vi "SDCP SMF Receiver and Transmitter - SMF Rx Table.vi"(2 "error in (no error)":errorcluster, 3 "Table reference":refnum<vi>) -> (0 "error out":errorcluster)   [LabVIEW 2020]
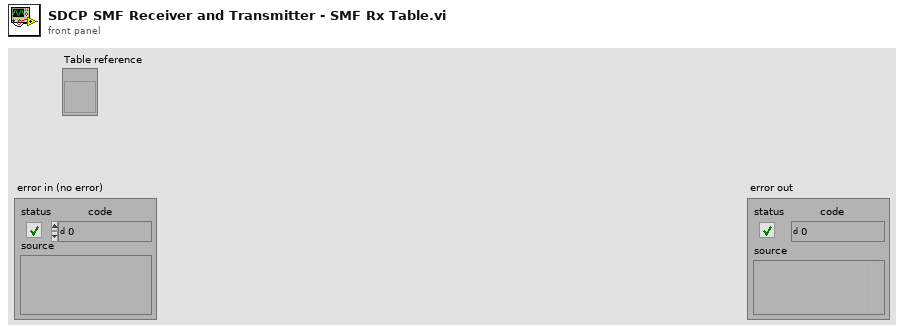
[diagram p1: front panel]
types:
  T1 = typedef "SDCP SMF Receiver and Transmitter - Notifier and Queues.ctl" = cluster{"Trace Queue":refnum<queue>, "Tx - Log Table Queue":refnum<queue>, "Tx - User Queue":refnum<queue>, "Rx - Log Table Queue":refnum<queue>, "Rx - User Queue":refnum<queue>, "Log status Notifier":refnum<notifier>, "Plot Queue":refnum<queue>}
  T2 = typedef "SDCP SMF logger - SMF with timestamp.ctl" = cluster{"Bytes":u8[], "Checksum":bool, "Time (ms)":u32, "Tx/Rx":string}
  T3 = typedef "SDCP - SMF parameter descriptors.ctl" = cluster{"Frame name":string, "Frame ID":i32, "Data type":string, "Start Position":i32, "Length":i32, "Factor":dbl, "Offset":dbl, "Parameter name":string, "Value":string}
  T4 = typedef "SDCP - Log Table - Element.ctl" = cluster{"Data frame":u8[], "Cycle time (ms)":i32, "Count":i32, "Frame ID":i32, "Frame name":string, "Parameter names":string[], "Parameter values":string[]}
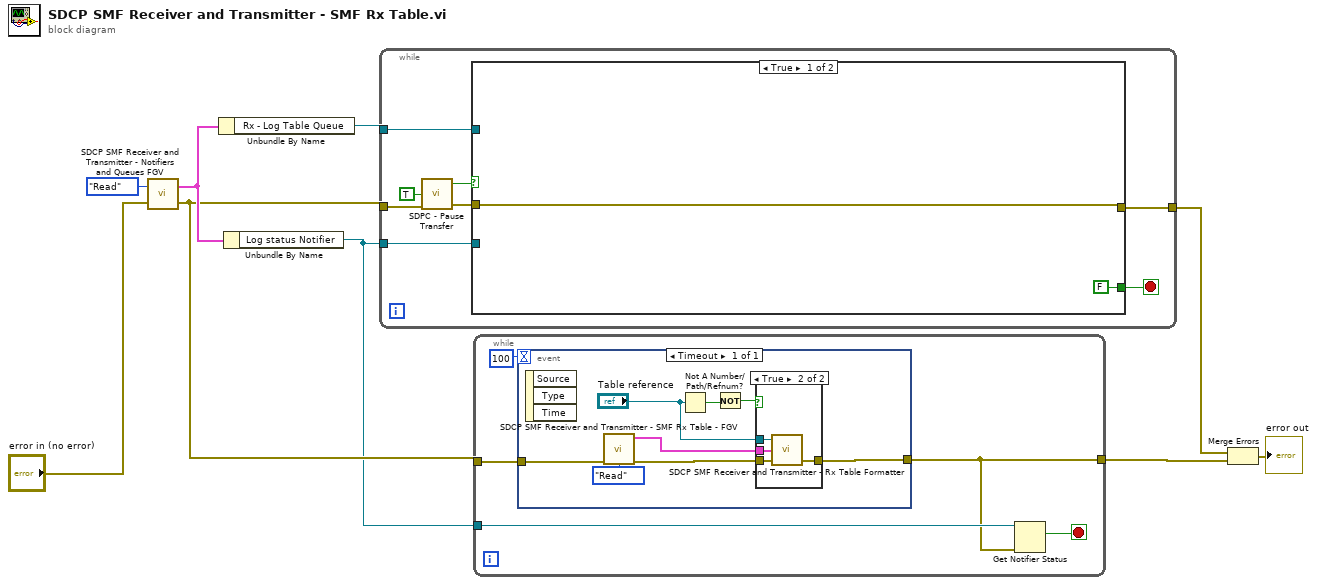
[diagram p0: block diagram]
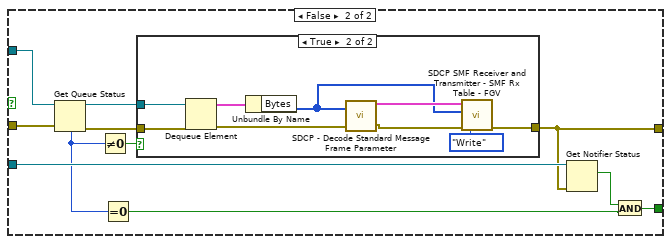
[diagram p3: hidden frame]
diagram:
  n1 = call "SDCP SMF Receiver and Transmitter - Notifiers and Queues FGV.vi"("error in (no error)"="error in (no error)", "Command"=enum16{"Initialize", "Read", "Deinitialize"}."Read") -> ("error out"=w3:errorcluster, "Output"=w6:T1)
  n2 = Unbundle By Name(w6) -> ("Rx - Log Table Queue"=w7:refnum<queue>)
  n3 = Unbundle By Name(w6) -> ("Log status Notifier"=w1:refnum<notifier>)
  n4 = while {
    tunnel: w3 -> [w13]
    tunnel: w7 -> [w15]
    tunnel: w1 -> [w17]
    tunnel: [w16] -> w5
    stop <- w14 stop-if-true
    n5 = call "SDPC - Pause Transfer.vi"("error in (no error)"=w13, "RD/nWR"=TRUE) -> ("error out"=w11:errorcluster, "Transfer paused"=w10:bool)  [unwired: 2 in]
    n6 = case shown="True" w10 {
      tunnel: w17 -> [_ w30]
      tunnel: [w19 w29] -> w16
      tunnel: w15 -> [_ w26]
      tunnel: [FALSE w23] -> w14
      tunnel: w11 -> [w19 w20]
      frame True {
      }
      frame False {
        n7 = Get Queue Status(queue=w26, error in (no error)=w20) -> (queue out=w25:refnum<queue>, error out=w28:errorcluster, # elements in queue=w22:i32)  [unwired: 1 in, 5 out]
        n8 = Not Equal To 0?(x=w22) -> (x != 0?=w27:bool)
        n9 = Equal To 0?(x=w22) -> (x = 0?=w21:bool)
        n10 = case shown="True" w27 {
          tunnel: [w31 w34] -> w29
          tunnel: w28 -> [w31 w33]
          tunnel: w25 -> [_ w32]
          frame False {
          }
          frame True {
            n11 = Dequeue Element(queue=w32, error in (no error)=w33) -> (element=w39:T2, error out=w40:errorcluster)  [unwired: 1 in, 2 out]
            n12 = Unbundle By Name(w39) -> ("Bytes"=w36:u8[])
            n13 = call "SDCP - Decode Standard Message Frame Parameter.vi"("error in (no error)"=w40, "Bytes in"=w36) -> ("error out"=w38:errorcluster, "SMF Parameters out"=w37:T3[])
            n14 = call "SDCP SMF Receiver and Transmitter - SMF Rx Table - FGV.vi"("error in (no error)"=w38, "Command"=enum16{"Reset", "Write", "Read"}."Write", "Bytes in"=w36, "Parameter descriptors"=w37) -> ("error out"=w34:errorcluster)  [unwired: 6 in, 1 out]
          }
        }
        n15 = Get Notifier Status(notifier=w30, error in (no error)=w29) -> (current notification=w24:bool)  [unwired: 4 out]
        n16 = And(x=w24, y=w21) -> (x .and. y?=w23:bool)
      }
    }
  }
  n17 = while {
    tunnel: w3 -> [w43]
    tunnel: [w41] -> w2
    tunnel: w1 -> [w44]
    stop <- w42 stop-if-true
    n18 = event shown="[0] Timeout" {
      selector: _ -> [_]
      dyn-events: _ -> [_]
      timeout: 100 -> [_]
      tunnel: w43 -> [w53]
      tunnel: [w47] -> w41
      event Timeout {
        n19 = event-data() -> ()  [unwired: 1 in, 3 out]
        n20 = call "SDCP SMF Receiver and Transmitter - SMF Rx Table - FGV.vi"("error in (no error)"=w53, "Command"=enum16{"Reset", "Write", "Read"}."Read") -> ("error out"=w51:errorcluster, "Elements of log table"=w50:T4[])  [unwired: 8 in]
        n21 = Not A Number/Path/Refnum?(number/path/refnum="Table reference") -> (NaN/Path/Refnum?=w49:bool)
        n22 = Not(x=w49) -> (.not. x?=w48:bool)
        n23 = case shown="True" w48 {
          tunnel: w51 -> [w54 w58]
          tunnel: w50 -> [_ w57]
          tunnel: [w54 w56] -> w47
          tunnel: "Table reference" -> [_ w55]
          frame False {
          }
          frame True {
            n24 = call "SDCP SMF Receiver and Transmitter - Rx Table Formatter.vi"("error in (no error)"=w58, "Elements of table"=w57, "Table reference"=w55) -> ("error out"=w56:errorcluster)  [unwired: 2 in]
          }
        }
      }
    }
    n25 = Get Notifier Status(notifier=w44, error in (no error)=w41) -> (current notification=w42:bool)  [unwired: 4 out]
  }
  n26 = Merge Errors(w5, w2) -> (→"error out":errorcluster)
